vi "FGV Zustandsbeleuchtung schalten.vi"(2 "Blinkgeschwindigkeit in ms":i32=300, 5 "Aufheizphase":i16, 11 "error in (no error)":errorcluster caption="Fehler (Eingang, kein Fehler)", 13 "Aktion":T1) -> (4 "Aufheizphase":bool, 15 "error out":errorcluster caption="Fehler (Ausgang)")   [LabVIEW 2020, in "Allgemein.lvlib"]
uses:
  Allgemein.lvlib
  Aktion FGV Zustandsbeleuchtung schalten.ctl
  FGV Zustaende Aktionen.ctl
  Funktionstasten/Zustaende.ctl
  Stoermeldungen/FGV Stoerungen Aktionen.ctl
  FGV Komm Status Aktionen.ctl
  Verwaltung/FGV OUT Aktionen.ctl
  Funktionstasten/Funktionstasten.lvlib
  Verwaltung/Verwaltung - cRIO.lvlib
  Stoermeldungen/Stoermeldungen.lvlib
  Kommunikation mit PC.lvlib
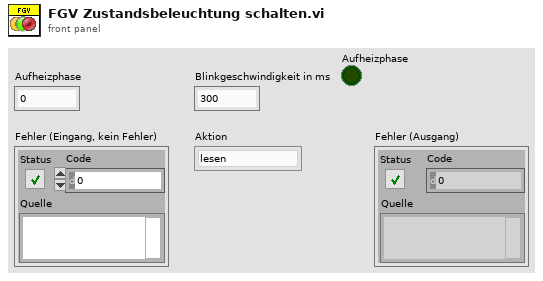
[diagram p1: front panel]
types:
  T1 = typedef "Allgemein.lvlib/Aktion FGV Zustandsbeleuchtung schalten.ctl" = enum16{"lesen", "prüfen", "init", "Bit löschen", "ansteuern", "Aufheizphase"}
  T2 = typedef "Allgemein.lvlib/FGV Zustaende Aktionen.ctl" = enum16{"lesen", "Zustand PC", "Zustand cRIO", "Bildnummer", "Samplepoint", "Sysloglevel"}
  T3 = typedef "Funktionstasten.lvlib/Zustaende.ctl" = enum16{"Standby", "Pause", "Eco", "Messen", "Kalibrieren", "Spülen Filter", "Spülen Leitung", "Umgebungsluft", "0-Gas", "Cal-Gas", "CG zu PNS", "-------------", "Init 1", "Init 2", "Init 3", "Init 4", "Messen vorbereiten", "Messen durchführen", "Exit"}
  T4 = typedef "Kommunikation mit PC.lvlib/FGV Komm Status Aktionen.ctl" = enum16{"lesen", "lebt PC?"}
  T5 = typedef "Stoermeldungen.lvlib/FGV Stoerungen Aktionen.ctl" = enum16{"lesen", "Störung aktiv?", "1-64", "65-128"}
  T6 = typedef "Verwaltung - cRIO.lvlib/FGV OUT Aktionen.ctl" = enum16{"lesen", "ANA OUT", "DO 0-31", "DO 32-47"}
  T7 = typedef "Verwaltung - cRIO.lvlib/Digital Ausgaenge 32-63.ctl" = cluster{"O32: Messgaspumpe EIN":bool, "O33: (Umgebungsluftpumpe)":bool, "O34: (Kondensatpumpe GK)":bool, "O35: Klima/Lüfter EIN":bool, "O36: Versorgung Heizungen":bool, "O37: Versorgung Heizungen":bool, "O38: (Gaskühler EIN (Freigabe))":bool, "O39: Störung FAS LP":bool, "O40: (Heizung Filterblock)":bool, "O41: Heizung HL zu FT-IR":bool, "O42: Heizung HL Extern SP1":bool, "O43: Heizung HL Extern SP2":bool, "O44: Heizung Reserve":bool, "O45: Heizung Reserve":bool, "O46: Statusbeleuchtung grün":bool, "O47: Statusbeleuchtung rot":bool}
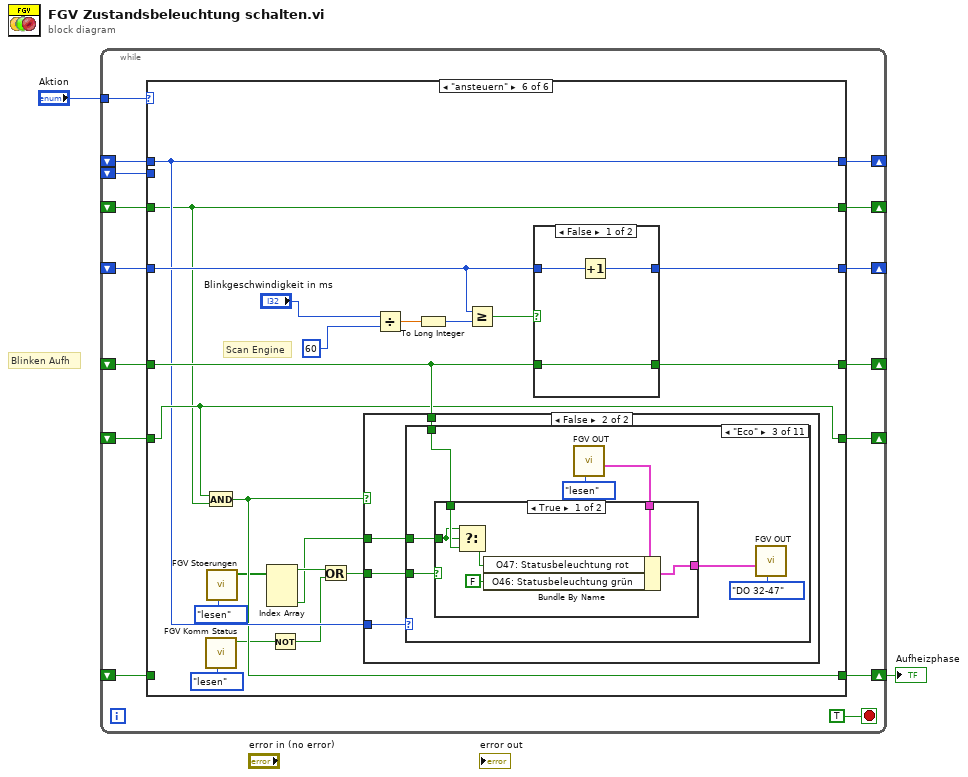
[diagram p0: block diagram]
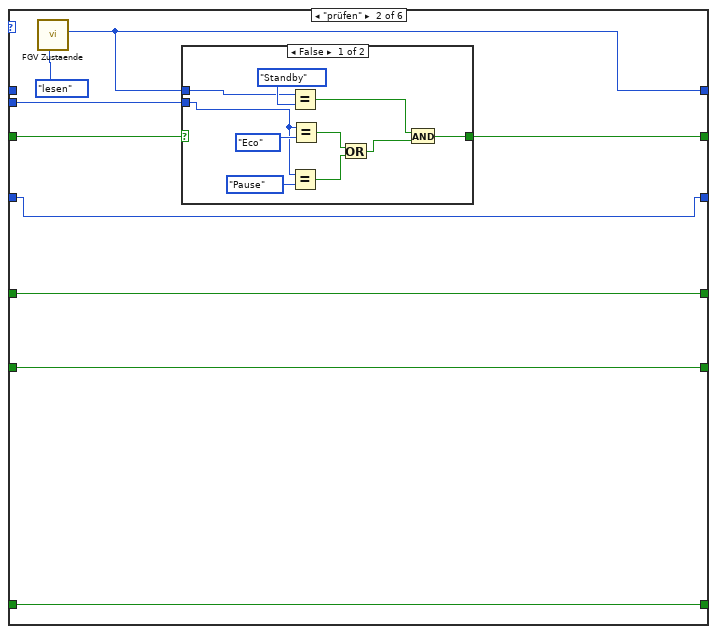
[diagram p3: hidden frame]
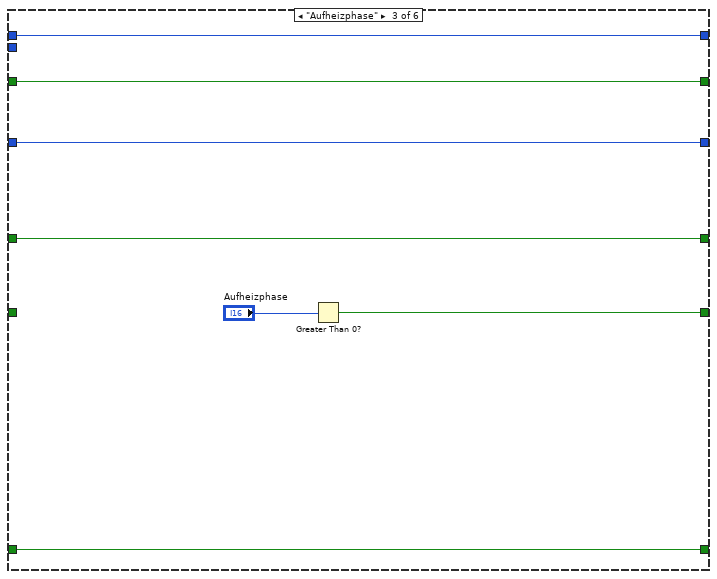
[diagram p5: hidden frame]
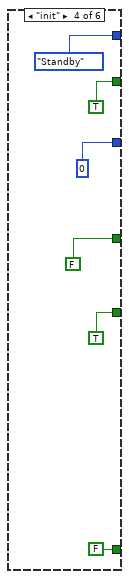
[diagram p6: hidden frame]
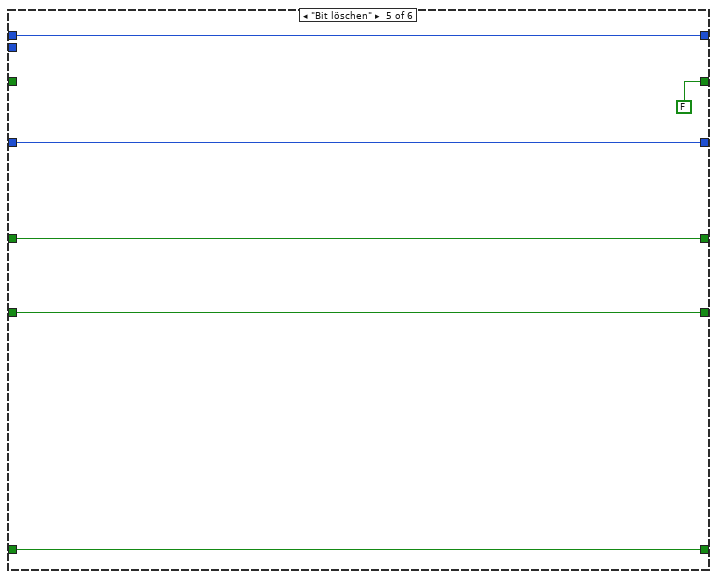
[diagram p7: hidden frame]
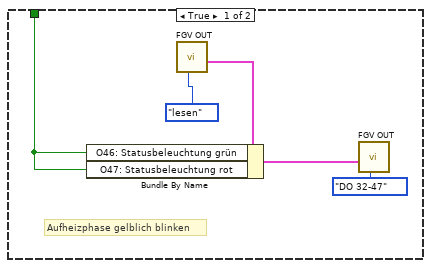
[diagram p8: hidden frame]
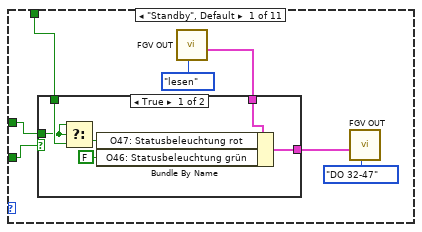
[diagram p9: hidden frame]
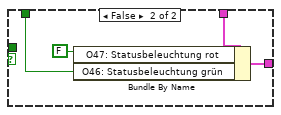
[diagram p10: hidden frame]
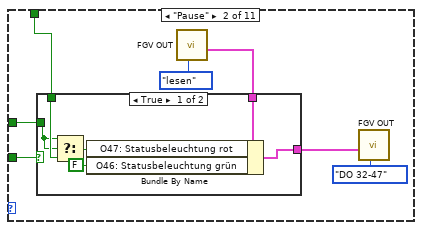
[diagram p11: hidden frame]
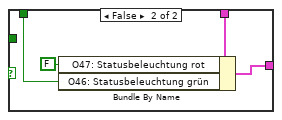
[diagram p12: hidden frame]
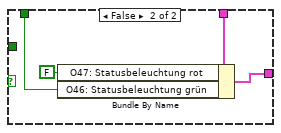
[diagram p13: hidden frame]
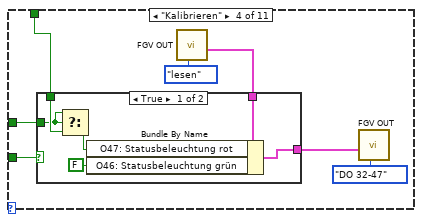
[diagram p14: hidden frame]
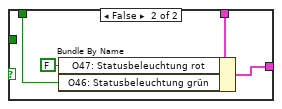
[diagram p15: hidden frame]
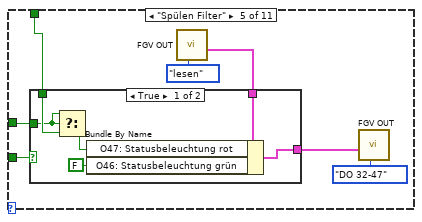
[diagram p16: hidden frame]
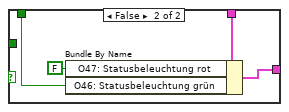
[diagram p17: hidden frame]
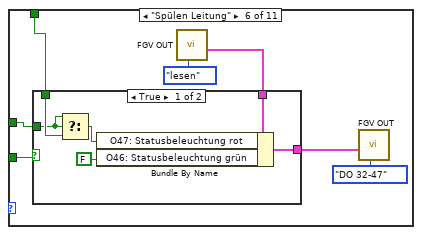
[diagram p18: hidden frame]
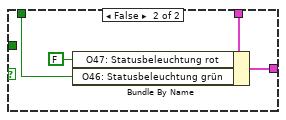
[diagram p19: hidden frame]
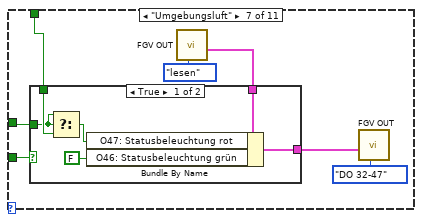
[diagram p20: hidden frame]
diagram:
  # "Blinken Aufh"
  n1 = while {
    shift-right: [w15] -> _
    shift-left: _ -> [w14]
    shift-left: _ -> [w13]
    tunnel: "Aktion" -> [w16]
    shift-right: [w12] -> _
    shift-left: _ -> [w11]
    shift-right: [w10] -> _
    shift-left: _ -> [w9]
    shift-right: [w8] -> _
    shift-left: _ -> [w7]
    shift-right: [w6] -> _
    shift-left: _ -> [w5]
    shift-right: [w4] -> w1
    shift-left: _ -> [w3]
    stop <- TRUE stop-if-true
    n2 = case shown="\"ansteuern\"" w16 {
      tunnel: [w23 w24 w50 Zustaende."Standby" ("Zustand cRIO") w62 w72] -> w15
      tunnel: w14 -> [w23 _ w50 _ w62 w72]
      tunnel: w13 -> [_ w31 _ _ _ _]
      tunnel: [w22 w28 w45 TRUE FALSE w71] -> w12
      tunnel: w11 -> [w22 w27 w45 _ _ w71]
      tunnel: [w21 w30 w49 0 w61 w80] -> w10
      tunnel: w9 -> [w21 w30 w49 _ w61 w79]
      tunnel: [w20 w29 w48 FALSE w59 w76] -> w8
      tunnel: w7 -> [w20 w29 w48 _ w59 w75]
      tunnel: [w19 w26 w46 TRUE w60 w74] -> w6
      tunnel: w5 -> [w19 w26 _ _ w60 w74]
      tunnel: [w18 w25 w44 FALSE w57 w70] -> w4
      tunnel: w3 -> [w18 w25 w44 _ w57 _]
      frame "lesen", Default {
      }
      frame "prüfen" {
        n3 = call "FGV Zustaende.vi"("Aktionen"=FGV_Zustaende_Aktionen."lesen") -> ("Zustand cRIO"=w24:T3)  [unwired: 6 in, 4 out]
        n4 = case shown="False" w27 {
          selector: w27 -> [_ w43]
          tunnel: w24 -> [w34 _]
          tunnel: w31 -> [w33 _]
          tunnel: [w35 w43] -> w28
          frame False {
            n5 = Equal?(x=w34, y=Zustaende."Standby") -> (x = y?=w36:bool)
            n6 = Equal?(x=w33, y=Zustaende."Pause") -> (x = y?=w38:bool)
            n7 = Equal?(x=w33, y=Zustaende."Eco") -> (x = y?=w39:bool)
            n8 = Or(x=w39, y=w38) -> (x .or. y?=w37:bool)
            n9 = And(x=w36, y=w37) -> (x .and. y?=w35:bool)
          }
          frame True {
          }
        }
      }
      frame "Aufheizphase" {
        n10 = Greater Than 0?(x="Aufheizphase") -> (x > 0?=w46:bool)
      }
      frame "init" {
      }
      frame "Bit löschen" {
      }
      frame "ansteuern" {
        # "Scan Engine"
        n11 = And(x=w74, y=w71) -> (x .and. y?=w70:bool)
        n12 = call "FGV Komm Status.vi"("Aktionen"=FGV_Komm_Status_Aktionen."lesen") -> ("lebt PC?"=w66:bool)  [unwired: 10 in]
        n13 = call "FGV Stoerungen.vi"("Aktionen"=FGV_Stoerungen_Aktionen."lesen") -> ("Störung aktiv?"=w64:bool[])  [unwired: 8 in, 2 out]
        n14 = Index Array(array=w64) -> (element #1=w69:bool, element #3=w63:bool)  [unwired: 3 in, 1 out]
        n15 = Not(x=w66) -> (.not. x?=w65:bool)
        n16 = Or(x=w69, y=w65) -> (x .or. y?=w67:bool)
        n17 = case shown="False" w70 {
          tunnel: w75 -> [w84 w92]
          tunnel: w72 -> [_ w91]
          tunnel: w67 -> [_ w90]
          tunnel: w63 -> [_ w89]
          frame True {
            # "Aufheizphase gelblich blinken"
            n18 = call "FGV OUT.vi"("Aktion"=FGV_OUT_Aktionen."lesen") -> ("DO 32-63"=w86:T7)  [unwired: 7 in, 3 out]
            n19 = Bundle By Name(cluster=w86, "O46: Statusbeleuchtung grün"=w84, "O47: Statusbeleuchtung rot"=w84) -> (w85:T7)
            n20 = call "FGV OUT.vi"("Aktion"=FGV_OUT_Aktionen."DO 32-47", "DO 32-63"=w85) -> ()  [unwired: 6 in, 4 out]
          }
          frame False {
            n21 = case shown="\"Eco\"" w91 {
              tunnel: w92 -> [w94 w111 w128 w145 w162 w179 w196 w213 w230 w247 w264]
              tunnel: w90 -> [w95 w112 w129 w146 w163 w180 w197 w214 w231 w248 w265]
              tunnel: w89 -> [w93 w110 w127 w144 w161 w178 w195 w212 w229 w246 w263]
              frame "Standby", Default {
                n22 = call "FGV OUT.vi"("Aktion"=FGV_OUT_Aktionen."lesen") -> ("DO 32-63"=w97:T7)  [unwired: 7 in, 3 out]
                n23 = case shown="True" w95 {
                  tunnel: w97 -> [w105 w109]
                  tunnel: [w104 w108] -> w96
                  tunnel: w94 -> [w101 w107]
                  tunnel: w93 -> [w100 _]
                  frame True {
                    n24 = Select(t=w100, s=w100, f=w101) -> (s? t:f=w102:bool)
                    n25 = Bundle By Name(cluster=w105, "O47: Statusbeleuchtung rot"=w102, "O46: Statusbeleuchtung grün"=FALSE ("O47: Statusbeleuchtung grün")) -> (w104:T7)
                  }
                  frame False {
                    n26 = Bundle By Name(cluster=w109, "O47: Statusbeleuchtung rot"=FALSE ("O46: Statusbeleuchtung rot"), "O46: Statusbeleuchtung grün"=w107) -> (w108:T7)
                  }
                }
                n27 = call "FGV OUT.vi"("Aktion"=FGV_OUT_Aktionen."DO 32-47", "DO 32-63"=w96) -> ()  [unwired: 6 in, 4 out]
              }
              frame "Pause" {
                n28 = call "FGV OUT.vi"("Aktion"=FGV_OUT_Aktionen."lesen") -> ("DO 32-63"=w114:T7)  [unwired: 7 in, 3 out]
                n29 = case shown="True" w112 {
                  tunnel: w114 -> [w122 w126]
                  tunnel: [w121 w125] -> w113
                  tunnel: w111 -> [w118 w124]
                  tunnel: w110 -> [w117 _]
                  frame True {
                    n30 = Select(t=w117, s=w117, f=w118) -> (s? t:f=w119:bool)
                    n31 = Bundle By Name(cluster=w122, "O47: Statusbeleuchtung rot"=w119, "O46: Statusbeleuchtung grün"=FALSE ("O47: Statusbeleuchtung grün")) -> (w121:T7)
                  }
                  frame False {
                    n32 = Bundle By Name(cluster=w126, "O47: Statusbeleuchtung rot"=FALSE ("O46: Statusbeleuchtung rot"), "O46: Statusbeleuchtung grün"=w124) -> (w125:T7)
                  }
                }
                n33 = call "FGV OUT.vi"("Aktion"=FGV_OUT_Aktionen."DO 32-47", "DO 32-63"=w113) -> ()  [unwired: 6 in, 4 out]
              }
              frame "Eco" {
                n34 = call "FGV OUT.vi"("Aktion"=FGV_OUT_Aktionen."lesen") -> ("DO 32-63"=w131:T7)  [unwired: 7 in, 3 out]
                n35 = case shown="True" w129 {
                  tunnel: w131 -> [w139 w143]
                  tunnel: [w138 w142] -> w130
                  tunnel: w128 -> [w135 w141]
                  tunnel: w127 -> [w134 _]
                  frame True {
                    n36 = Select(t=w134, s=w134, f=w135) -> (s? t:f=w136:bool)
                    n37 = Bundle By Name(cluster=w139, "O47: Statusbeleuchtung rot"=w136, "O46: Statusbeleuchtung grün"=FALSE ("O47: Statusbeleuchtung grün")) -> (w138:T7)
                  }
                  frame False {
                    n38 = Bundle By Name(cluster=w143, "O47: Statusbeleuchtung rot"=FALSE ("O46: Statusbeleuchtung rot"), "O46: Statusbeleuchtung grün"=w141) -> (w142:T7)
                  }
                }
                n39 = call "FGV OUT.vi"("Aktion"=FGV_OUT_Aktionen."DO 32-47", "DO 32-63"=w130) -> ()  [unwired: 6 in, 4 out]
              }
              frame "Kalibrieren" {
                n40 = call "FGV OUT.vi"("Aktion"=FGV_OUT_Aktionen."lesen") -> ("DO 32-63"=w148:T7)  [unwired: 7 in, 3 out]
                n41 = case shown="True" w146 {
                  tunnel: w148 -> [w156 w160]
                  tunnel: [w155 w159] -> w147
                  tunnel: w145 -> [w152 w158]
                  tunnel: w144 -> [w151 _]
                  frame True {
                    n42 = Select(t=w151, s=w151, f=w152) -> (s? t:f=w153:bool)
                    n43 = Bundle By Name(cluster=w156, "O47: Statusbeleuchtung rot"=w153, "O46: Statusbeleuchtung grün"=FALSE ("O47: Statusbeleuchtung grün")) -> (w155:T7)
                  }
                  frame False {
                    n44 = Bundle By Name(cluster=w160, "O47: Statusbeleuchtung rot"=FALSE ("O46: Statusbeleuchtung rot"), "O46: Statusbeleuchtung grün"=w158) -> (w159:T7)
                  }
                }
                n45 = call "FGV OUT.vi"("Aktion"=FGV_OUT_Aktionen."DO 32-47", "DO 32-63"=w147) -> ()  [unwired: 6 in, 4 out]
              }
              frame "Spülen Filter" {
                n46 = call "FGV OUT.vi"("Aktion"=FGV_OUT_Aktionen."lesen") -> ("DO 32-63"=w165:T7)  [unwired: 7 in, 3 out]
                n47 = case shown="True" w163 {
                  tunnel: w165 -> [w173 w177]
                  tunnel: [w172 w176] -> w164
                  tunnel: w162 -> [w169 w175]
                  tunnel: w161 -> [w168 _]
                  frame True {
                    n48 = Select(t=w168, s=w168, f=w169) -> (s? t:f=w170:bool)
                    n49 = Bundle By Name(cluster=w173, "O47: Statusbeleuchtung rot"=w170, "O46: Statusbeleuchtung grün"=FALSE ("O47: Statusbeleuchtung grün")) -> (w172:T7)
                  }
                  frame False {
                    n50 = Bundle By Name(cluster=w177, "O47: Statusbeleuchtung rot"=FALSE ("O46: Statusbeleuchtung rot"), "O46: Statusbeleuchtung grün"=w175) -> (w176:T7)
                  }
                }
                n51 = call "FGV OUT.vi"("Aktion"=FGV_OUT_Aktionen."DO 32-47", "DO 32-63"=w164) -> ()  [unwired: 6 in, 4 out]
              }
              frame "Spülen Leitung" {
                n52 = call "FGV OUT.vi"("Aktion"=FGV_OUT_Aktionen."lesen") -> ("DO 32-63"=w182:T7)  [unwired: 7 in, 3 out]
                n53 = case shown="True" w180 {
                  tunnel: w182 -> [w190 w194]
                  tunnel: [w189 w193] -> w181
                  tunnel: w179 -> [w186 w192]
                  tunnel: w178 -> [w185 _]
                  frame True {
                    n54 = Select(t=w185, s=w185, f=w186) -> (s? t:f=w187:bool)
                    n55 = Bundle By Name(cluster=w190, "O47: Statusbeleuchtung rot"=w187, "O46: Statusbeleuchtung grün"=FALSE ("O47: Statusbeleuchtung grün")) -> (w189:T7)
                  }
                  frame False {
                    n56 = Bundle By Name(cluster=w194, "O47: Statusbeleuchtung rot"=FALSE ("O46: Statusbeleuchtung rot"), "O46: Statusbeleuchtung grün"=w192) -> (w193:T7)
                  }
                }
                n57 = call "FGV OUT.vi"("Aktion"=FGV_OUT_Aktionen."DO 32-47", "DO 32-63"=w181) -> ()  [unwired: 6 in, 4 out]
              }
              frame "Umgebungsluft" {
                n58 = call "FGV OUT.vi"("Aktion"=FGV_OUT_Aktionen."lesen") -> ("DO 32-63"=w199:T7)  [unwired: 7 in, 3 out]
                n59 = case shown="True" w197 {
                  tunnel: w199 -> [w207 w211]
                  tunnel: [w206 w210] -> w198
                  tunnel: w196 -> [w203 w209]
                  tunnel: w195 -> [w202 _]
                  frame True {
                    n60 = Select(t=w202, s=w202, f=w203) -> (s? t:f=w204:bool)
                    n61 = Bundle By Name(cluster=w207, "O47: Statusbeleuchtung rot"=w204, "O46: Statusbeleuchtung grün"=FALSE ("O47: Statusbeleuchtung grün")) -> (w206:T7)
                  }
                  frame False {
                    n62 = Bundle By Name(cluster=w211, "O47: Statusbeleuchtung rot"=FALSE ("O46: Statusbeleuchtung rot"), "O46: Statusbeleuchtung grün"=w209) -> (w210:T7)
                  }
                }
                n63 = call "FGV OUT.vi"("Aktion"=FGV_OUT_Aktionen."DO 32-47", "DO 32-63"=w198) -> ()  [unwired: 6 in, 4 out]
              }
              frame "0-Gas" {
                n64 = call "FGV OUT.vi"("Aktion"=FGV_OUT_Aktionen."lesen") -> ("DO 32-63"=w216:T7)  [unwired: 7 in, 3 out]
                n65 = case shown="True" w214 {
                  tunnel: w216 -> [w224 w228]
                  tunnel: [w223 w227] -> w215
                  tunnel: w213 -> [w220 w226]
                  tunnel: w212 -> [w219 _]
                  frame True {
                    n66 = Select(t=w219, s=w219, f=w220) -> (s? t:f=w221:bool)
                    n67 = Bundle By Name(cluster=w224, "O47: Statusbeleuchtung rot"=w221, "O46: Statusbeleuchtung grün"=FALSE ("O47: Statusbeleuchtung grün")) -> (w223:T7)
                  }
                  frame False {
                    n68 = Bundle By Name(cluster=w228, "O47: Statusbeleuchtung rot"=FALSE ("O46: Statusbeleuchtung rot"), "O46: Statusbeleuchtung grün"=w226) -> (w227:T7)
                  }
                }
                n69 = call "FGV OUT.vi"("Aktion"=FGV_OUT_Aktionen."DO 32-47", "DO 32-63"=w215) -> ()  [unwired: 6 in, 4 out]
              }
              frame "Cal-Gas" {
                n70 = call "FGV OUT.vi"("Aktion"=FGV_OUT_Aktionen."lesen") -> ("DO 32-63"=w233:T7)  [unwired: 7 in, 3 out]
                n71 = case shown="True" w231 {
                  tunnel: w233 -> [w241 w245]
                  tunnel: [w240 w244] -> w232
                  tunnel: w230 -> [w237 w243]
                  tunnel: w229 -> [w236 _]
                  frame True {
                    n72 = Select(t=w236, s=w236, f=w237) -> (s? t:f=w238:bool)
                    n73 = Bundle By Name(cluster=w241, "O47: Statusbeleuchtung rot"=w238, "O46: Statusbeleuchtung grün"=FALSE ("O47: Statusbeleuchtung grün")) -> (w240:T7)
                  }
                  frame False {
                    n74 = Bundle By Name(cluster=w245, "O47: Statusbeleuchtung rot"=FALSE ("O46: Statusbeleuchtung rot"), "O46: Statusbeleuchtung grün"=w243) -> (w244:T7)
                  }
                }
                n75 = call "FGV OUT.vi"("Aktion"=FGV_OUT_Aktionen."DO 32-47", "DO 32-63"=w232) -> ()  [unwired: 6 in, 4 out]
              }
              frame "CG zu PNS" {
                n76 = call "FGV OUT.vi"("Aktion"=FGV_OUT_Aktionen."lesen") -> ("DO 32-63"=w250:T7)  [unwired: 7 in, 3 out]
                n77 = case shown="True" w248 {
                  tunnel: w250 -> [w258 w262]
                  tunnel: [w257 w261] -> w249
                  tunnel: w247 -> [w254 w260]
                  tunnel: w246 -> [w253 _]
                  frame True {
                    n78 = Select(t=w253, s=w253, f=w254) -> (s? t:f=w255:bool)
                    n79 = Bundle By Name(cluster=w258, "O47: Statusbeleuchtung rot"=w255, "O46: Statusbeleuchtung grün"=FALSE ("O47: Statusbeleuchtung grün")) -> (w257:T7)
                  }
                  frame False {
                    n80 = Bundle By Name(cluster=w262, "O47: Statusbeleuchtung rot"=FALSE ("O46: Statusbeleuchtung rot"), "O46: Statusbeleuchtung grün"=w260) -> (w261:T7)
                  }
                }
                n81 = call "FGV OUT.vi"("Aktion"=FGV_OUT_Aktionen."DO 32-47", "DO 32-63"=w249) -> ()  [unwired: 6 in, 4 out]
              }
              frame "Messen" {
                n82 = call "FGV OUT.vi"("Aktion"=FGV_OUT_Aktionen."lesen") -> ("DO 32-63"=w267:T7)  [unwired: 7 in, 3 out]
                n83 = case shown="True" w265 {
                  tunnel: w267 -> [w275 w279]
                  tunnel: [w274 w278] -> w266
                  tunnel: w264 -> [w271 _]
                  tunnel: w263 -> [w270 _]
                  frame True {
                    n84 = Select(t=w270, s=w270, f=w271) -> (s? t:f=w272:bool)
                    n85 = Bundle By Name(cluster=w275, "O47: Statusbeleuchtung rot"=w272, "O46: Statusbeleuchtung grün"=FALSE ("O47: Statusbeleuchtung grün")) -> (w274:T7)
                  }
                  frame False {
                    n86 = Bundle By Name(cluster=w279, "O46: Statusbeleuchtung grün"=TRUE ("O47: Statusbeleuchtung grün"), "O47: Statusbeleuchtung rot"=FALSE ("O46: Statusbeleuchtung rot")) -> (w278:T7)
                  }
                }
                n87 = call "FGV OUT.vi"("Aktion"=FGV_OUT_Aktionen."DO 32-47", "DO 32-63"=w266) -> ()  [unwired: 6 in, 4 out]
              }
            }
          }
        }
        n88 = Divide(x="Blinkgeschwindigkeit in ms", y=60) -> (x/y=w81:dbl)
        n89 = To Long Integer(number=w81) -> (32bit integer=w78:i32)
        n90 = Greater Or Equal?(x=w79, y=w78) -> (x >= y?=w77:bool)
        n91 = case shown="False" w77 {
          tunnel: w79 -> [w282 _]
          tunnel: [w281 0] -> w80
          tunnel: w75 -> [w280 w284]
          tunnel: [w280 w283] -> w76
          frame False {
            n92 = Increment(x=w282) -> (x+1=w281:i32)
          }
          frame True {
            n93 = Not(x=w284) -> (.not. x?=w283:bool)
          }
        }
      }
    }
  }
  "Aufheizphase" <- w1
